vi "PH_PowerUnit_BaseClass.Calc State PU.vi"(0 "i ref in":refnum<vi>, 5 "error in (no error)":errorcluster) -> (14 "i ref out":refnum<vi>, 19 "error out":errorcluster)   [LabVIEW 2014, in "PH_PowerUnit_BaseClass.lvlib"]
doc: "In this VI the state of the PU (running, failure or alarm) is calculated. Depending on the state, several things are done."
uses:
  PH_PowerUnit_BaseClass.lvlib
  PH_StatusHandler/PH_StatusHandler.lvlib
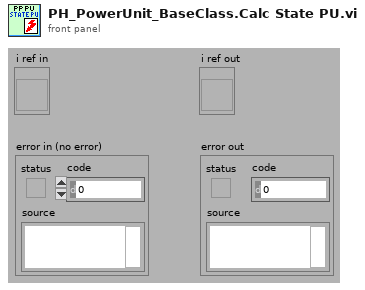
[diagram p1: front panel]
types:
  T1 = typedef "PH_StatusHandler.lvlib/PH_StatusHandler.Status.ctl" = i16
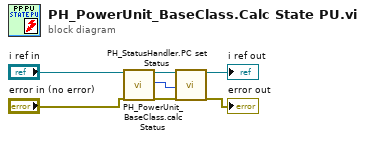
[diagram p0: block diagram]
diagram:
  n1 = call "PH_PowerUnit_BaseClass.calc Status.vi"("VI in"="i ref in", "error in (no error)"="error in (no error)") -> ("VI out"=w2:refnum<vi>, "PU Status"=w1:T1, "error out"=w3:errorcluster)  [unwired: 15 in]
  n2 = call "PH_StatusHandler.PC set Status.vi"("i ref in"=w2, "Status"=w1, "error in (no error)"=w3) -> ("i ref out"=→"i ref out":refnum<vi>, "error out"=→"error out":errorcluster)  [unwired: 15 in]
